vi "Start Post Processing.vi"(8 "error in (no error)":errorcluster, 9 "Open plot":bool, 10 "Result in":refnum<class "Acquired Result.lvclass">, 11 "Monitor-Pulse in":refnum<class "Application Controller.lvclass">) -> (0 "error out":errorcluster, 2 "Started":bool, 3 "Monitor-Pulse out":refnum<class "Application Controller.lvclass">)   [LabVIEW 2016, in "Application Controller.lvclass"]
uses:
  Application Controller.lvclass
  NHMFL_Core/Libraries/Instruments/Results/Acquired Result/Acquired Result.lvclass
  Application Controller.lvclass/Application Controller.ctl
  NHMFL_Core/Libraries/Queued Listbox/Queued Listbox.xctl
  Process Object Messages/Process Result Msg/Process Result Msg.lvclass/Process Result Msg.ctl
  <vilib>/ActorFramework/Message Enqueuer/Message Enqueuer.lvclass/Message Enqueuer.ctl
  <vilib>/ActorFramework/Message Enqueuer/Enqueue.vi
  Process Object Messages/Process Result Msg/Process Result Msg.lvclass
  C:/Program Files/National Instruments/LabVIEW 2016/vi.lib/ActorFramework/Message/Message.lvclass
  <vilib>/ActorFramework/Message Priority Queue/Priority Enqueue.vi
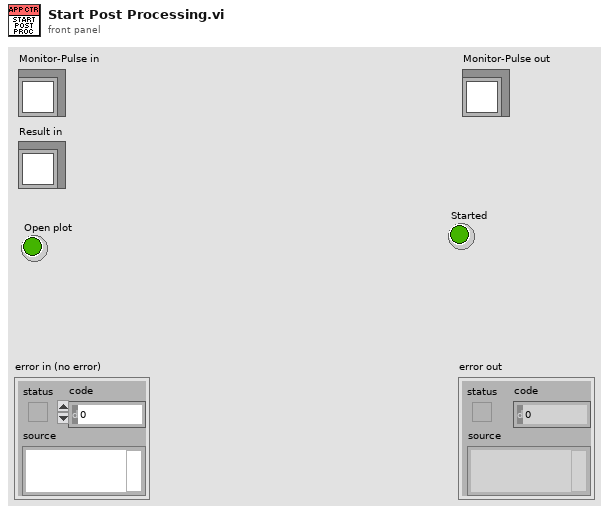
[diagram p1: front panel]
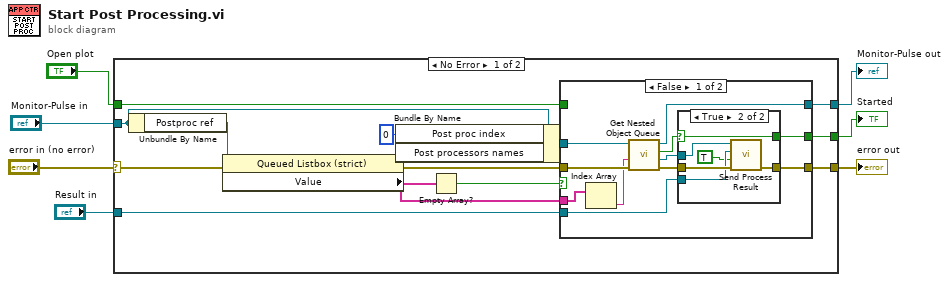
[diagram p0: block diagram]
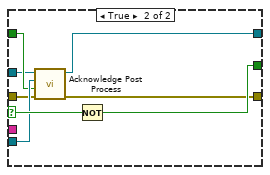
[diagram p3: hidden frame]
diagram:
  n1 = case shown="No Error" "error in (no error)" {
    selector: "error in (no error)" -> [w19 w49]
    tunnel: [w17 w49] -> w6
    tunnel: [w16 w48] -> w4
    tunnel: "Monitor-Pulse in" -> [w9 w48]
    tunnel: "Result in" -> [w14 _]
    tunnel: [w13 _] -> w2
    tunnel: "Open plot" -> [w12 _]
    frame No Error {
      n2 = Unbundle By Name(w9) -> ("Postproc ref"=w20:refnum<vi>)
      n3 = property class="Queued Listbox (strict)"(reference=w20, error in=w19) -> (error out=w18:errorcluster, "Value"=w11:string[])  [unwired: 1 out]
      n4 = Bundle By Name(cluster=w9, "Post proc index"=0, "Post processors names"=w11) -> (w8:refnum<class "Application Controller.lvclass">)
      n5 = Empty Array?(array=w11) -> (empty?=w15:bool)
      n6 = case shown="False" w15 {
        selector: w15 -> [_ w47]
        tunnel: w8 -> [w31 w40]
        tunnel: w11 -> [w22 _]
        tunnel: w18 -> [w24 w43]
        tunnel: [w23 w41] -> w17
        tunnel: [w26 w42] -> w16
        tunnel: w14 -> [w27 w45]
        tunnel: [w25 w46] -> w13
        tunnel: w12 -> [_ w44]
        frame False {
          n7 = Index Array(array=w22) -> (element=w21:string)  [unwired: 1 in]
          n8 = call-dynamic "Get Nested Object Queue.vi"("error in (no error)"=w24, "Name"=w21, "Measure Object in"=w31) -> ("error out"=w29:errorcluster, "Object Enqueuer"=w30:refnum<class "Message Enqueuer.lvclass">, "Found?"=w28:bool, "Measure Object out"=w26:refnum<class "Application Controller.lvclass">)  [unwired: 5 in]
          n9 = case shown="True" w28 {
            selector: w28 -> [w32 w34]
            tunnel: w30 -> [_ w39]
            tunnel: w29 -> [w33 w38]
            tunnel: [w33 w37] -> w23
            tunnel: w27 -> [_ w36]
            tunnel: [w32 w34] -> w25
            frame False {
            }
            frame True {
              n10 = call "Send Process Result.vi"("error in (no error)"=w38, "Acknowledge"=TRUE, "Result in"=w36, "Message Enqueuer"=w39) -> ("error out"=w37:errorcluster)  [unwired: 6 in, 1 out]
            }
          }
        }
        frame True {
          n11 = call-dynamic "Acknowledge Post Process.vi"("error in (no error)"=w43, "Open plot"=w44, "Ack Result"=w45, "Monitor-Pulse in"=w40) -> ("error out"=w41:errorcluster, "Monitor-Pulse out"=w42:refnum<class "Application Controller.lvclass">)  [unwired: 5 in, 1 out]
          n12 = Not(x=w47) -> (.not. x?=w46:bool)
        }
      }
    }
    frame Error {
    }
  }
  "error out" <- w6
  "Monitor-Pulse out" <- w4
  "Started" <- w2
